vi "Close Panel.vi"(8 "error in (no error)":errorcluster, 10 "Panel":refnum<class "Panel.lvclass">, 11 "PanelManager in":refnum<class "PanelManager.lvclass">) -> (0 "error out":errorcluster, 3 "PanelManager out":refnum<class "PanelManager.lvclass">)   [LabVIEW 2018, in "OOPanel.lvlib" / "PanelManager.lvclass"]
uses:
  PanelManager.lvclass
  Panel/Panel.lvclass
  PanelManager.lvclass/PanelManager.ctl
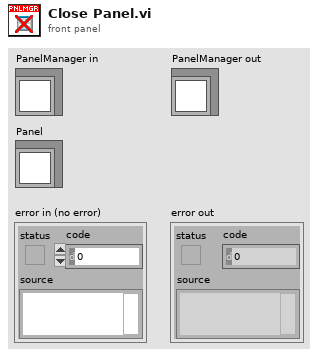
[diagram p1: front panel]
types:
  T1 = typedef "OOPanel.lvlib/PanelManager.lvclass/Ref Data.ctl" = cluster{"Panels":T2, "Subpanel Map":T3}
  T2 = typedef "OOPanel.lvlib/PanelManager.lvclass/Panels.ctl" = cluster{"Names":string[], "Instances":refnum<class "Panel.lvclass">[]}
  T3 = typedef "OOPanel.lvlib/PanelManager.lvclass/SubPanel Map.ctl" = cluster{"SubPanels":refnum<vi>[], "Panels":refnum<class "Panel.lvclass">[]}
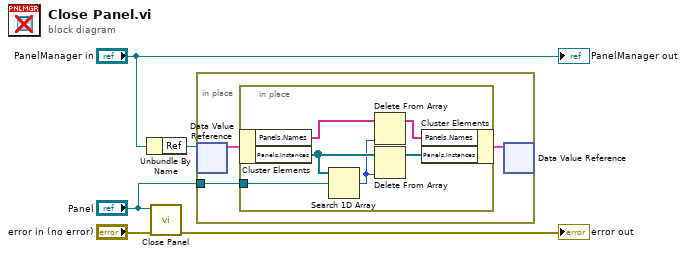
[diagram p0: block diagram]
diagram:
  n1 = Unbundle By Name("PanelManager in") -> ("Ref"=w3:refnum<data-value>)
  n2 = call "Close Panel.vi"("error in (no error)"="error in (no error)", "Panel in"="Panel") -> ("error out"=→"error out":errorcluster)  [unwired: 8 in, 1 out]
  n3 = in-place {
    in-place-border: "Panel" -> [w6]
    n4 = in-place-dvr #1(w3) -> (w8:T1)  [unwired: 1 out]
    n5 = in-place {
      in-place-border: w6 -> [w14]
      n6 = in-place-cluster #2(w8) -> ("Panels.Names"=w12:string[], "Panels.Instances"=w13:refnum<class "Panel.lvclass">[])
      n7 = Search 1D Array(1D array=w13, element=w14) -> (index of element=w11:i32)  [unwired: 1 in]
      n8 = Delete From Array(array=w12, index=w11) -> (array with subset deleted=w10:string[])  [unwired: 1 in, 1 out]
      n9 = Delete From Array(array=w13, index=w11) -> (array with subset deleted=w9:refnum<class "Panel.lvclass">[])  [unwired: 1 in, 1 out]
      n10 = in-place-cluster #2("Panels.Names"=w10, "Panels.Instances"=w9) -> (w7:T1)
    }
    n11 = in-place-dvr #1(w7) -> ()  [unwired: 2 out]
  }
  "PanelManager out" <- "PanelManager in"
